vi "motor_sensor.vi"() -> ()   [LabVIEW 2020]
panel:
  in  "VISA resource name":refnum<visa-resource-name>
  in  "Rotate":string
  in  "Forward Direction":string
  out "Range":string
  in  "OK Button":bool
  in  "byte count":u32
  in  "stop":bool
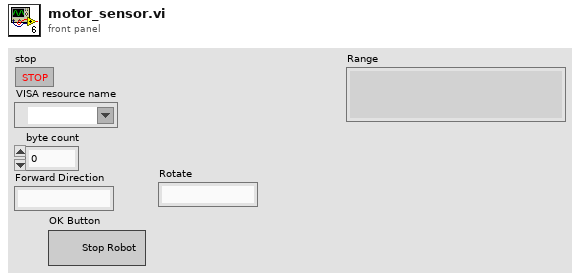
[diagram p1: front panel]
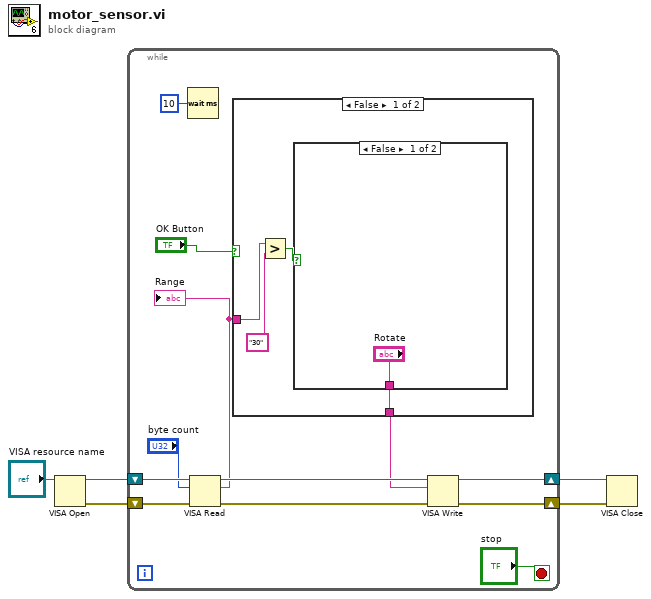
[diagram p0: block diagram]
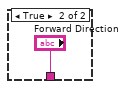
[diagram p2: hidden frame]
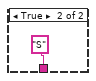
[diagram p3: hidden frame]
diagram:
  n1 = VISA Open(VISA resource name="VISA resource name") -> (VISA resource name=w5:refnum<visa-resource-name>, error out=w3:errorcluster)  [unwired: 4 in]
  n2 = while {
    shift-right: [w15] -> w4
    shift-left: w5 -> [w17]
    shift-right: [w12] -> w2
    shift-left: w3 -> [w14]
    stop <- "stop" stop-if-true
    n3 = Wait (ms)(milliseconds to wait=u32 10) -> ()  [unwired: 1 out]
    n4 = VISA Read(VISA resource name=w17, byte count="byte count", error in (no error)=w14) -> (VISA resource name out=w16:refnum<visa-resource-name>, read buffer=w6:string, error out=w13:errorcluster)  [unwired: 1 out]
    "Range" <- w6
    n5 = case shown="False" "OK Button" {
      tunnel: [w21 "S"] -> w8
      tunnel: w6 -> [w19 _]
      frame False {
        n6 = Greater?(x=w19, y="30") -> (0:w20:bool)
        n7 = case shown="False" w20 {
          tunnel: ["Rotate" "Forward Direction"] -> w21
          frame False {
          }
          frame True {
          }
        }
      }
      frame True {
      }
    }
    n8 = VISA Write(VISA resource name=w16, write buffer=w8, error in (no error)=w13) -> (VISA resource name out=w15:refnum<visa-resource-name>, error out=w12:errorcluster)  [unwired: 1 out]
  }
  n9 = VISA Close(VISA resource name=w4, error in (no error)=w2) -> ()  [unwired: 1 out]
